vi "Calc - FlowPPH.vi"(10 "02-05-9205":dbl[](array[numeric]), 11 "RhoFuel":dbl) -> (3 "FlowPPH":dbl)   [LabVIEW 2018, in "Controller (Host).lvlib"]
uses:
  Controller (Host).lvlib
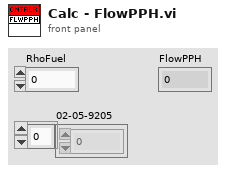
[diagram p1: front panel]
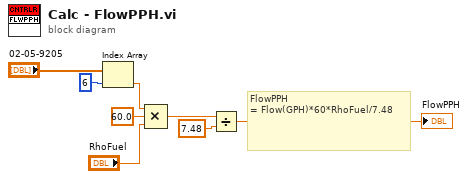
[diagram p0: block diagram]
diagram:
  # "FlowPPH\n= Flow(GPH)*60*RhoFuel/7.48"
  n1 = Index Array(array="02-05-9205", index=6) -> (element=w6:dbl)
  n2 = Compound Arithmetic op=MULTIPLY(w6, 60.0 ("value"), "RhoFuel") -> (w2:dbl)
  n3 = Divide(x=w2, y=7.48) -> (x/y=→"FlowPPH":dbl)
